vi "FromCaller.vi"(8 "error in (no error)":errorcluster, 9 "timeout in ms (-1)":i32=-1, 11 "JQMHStartup in":refnum<class "RQMHStartup.lvclass">) -> (0 "error out":errorcluster, 1 "Data":variant, 2 "Command":T1=enum."Error", 3 "JQMHStartup out":refnum<class "RQMHStartup.lvclass">)   [LabVIEW 2024, in "RQMHStartup.lvclass"]
uses:
  RQMHStartup.lvclass
  Command.ctl
  RQMHStartup.lvclass/RQMHStartup.ctl
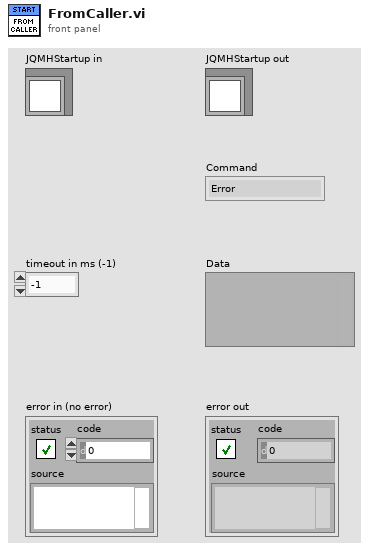
[diagram p1: front panel]
types:
  T1 = typedef "RQMHStartup.lvclass/Command.ctl" = enum16{"Default", "No Override", "Error", "ACK Created", "ACK Mod Reg", "ACK Caller Reg"}
  T2 = typedef "RQMHStartup.lvclass/Message.ctl" = cluster{"Command":T1, "Data":variant}
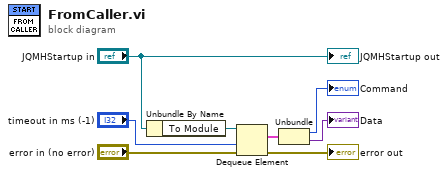
[diagram p0: block diagram]
diagram:
  n1 = Unbundle By Name("JQMHStartup in") -> ("To Module"=w2:refnum<queue>)
  n2 = Dequeue Element(queue=w2, timeout in ms (-1)="timeout in ms (-1)", error in (no error)="error in (no error)") -> (element=w1:T2, error out=→"error out":errorcluster)  [unwired: 2 out]
  n3 = Unbundle(w1) -> ("Command"=→"Command":T1, "Data"=→"Data":variant)
  "JQMHStartup out" <- "JQMHStartup in"
